vi "PRF_control.vi"(4 "PRF_Event Down":bool, 5 "mode selection":string(combo), 6 "error in (no error)":errorcluster, 7 "Input PRF":dbl, 8 "timeout (ms)":dbl=40000.0 format="%.2f", 9 "TCP from Orchid in":refnum<k5>) -> (0 "error out":errorcluster, 1 "PRF":dbl, 3 "connection ID out":refnum<k5>)   [LabVIEW 2016]
uses:
  TemperatureMeasure/Thermal_type.vi
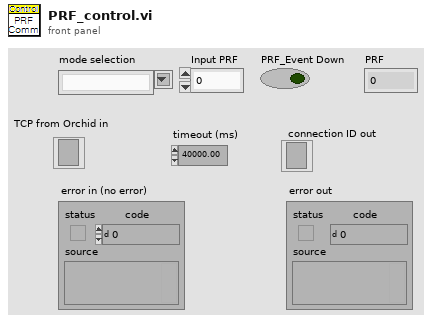
[diagram p1: front panel]
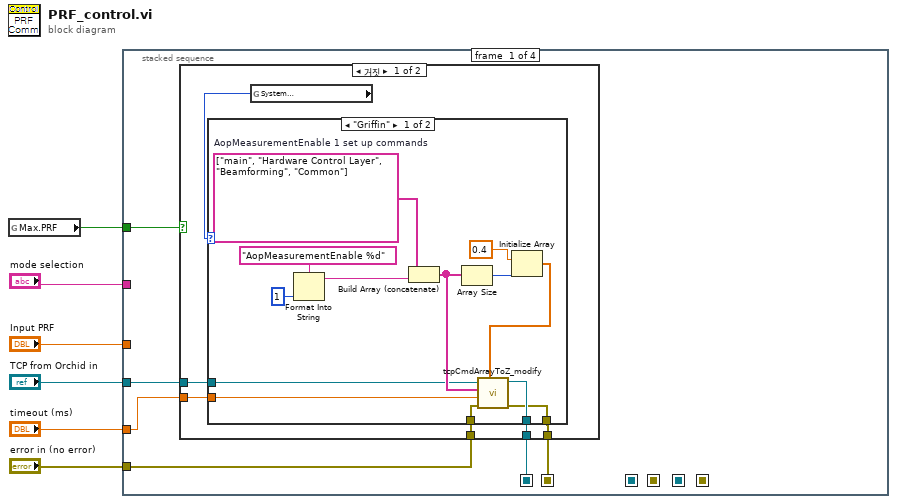
[diagram p0: block diagram]
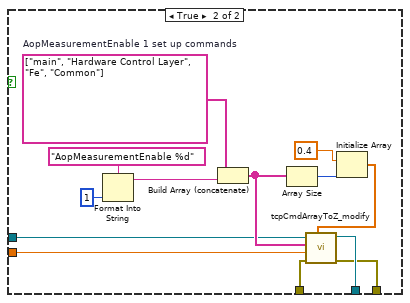
[diagram p3: hidden frame]
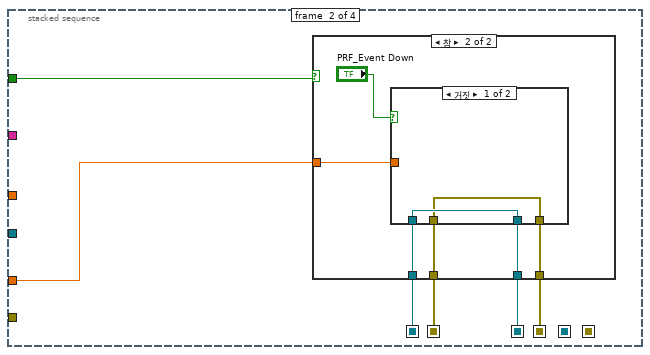
[diagram p4: hidden frame]
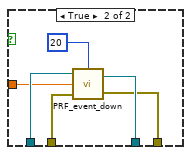
[diagram p6: hidden frame]
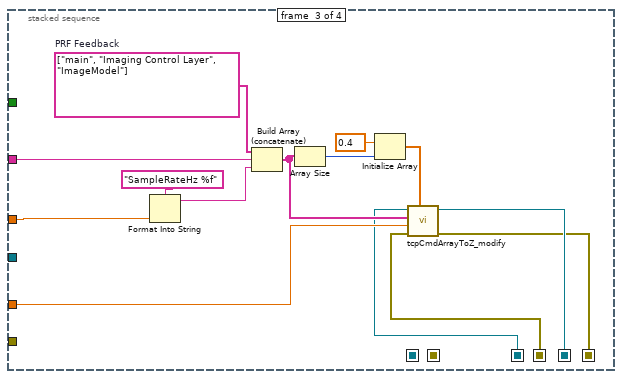
[diagram p7: hidden frame]
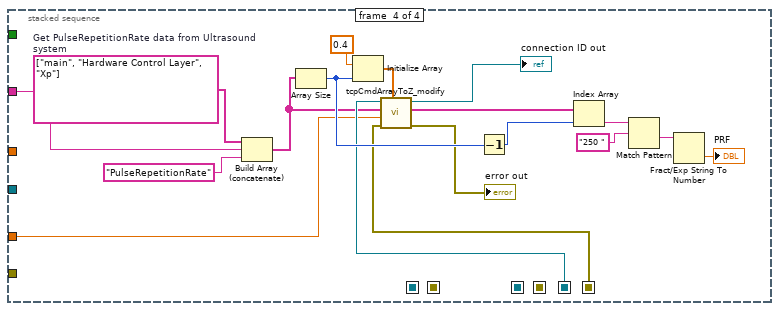
[diagram p8: hidden frame]
diagram:
  n1 = global read "Thermal_type.vi" "Max.PRF"() -> (w1:bool)
  n2 = stacked-sequence {
    seq-local: [w9 _ _ _] -> [_ w52 _ _]
    seq-local: [w8 _ _ _] -> [_ w51 _ _]
    seq-local: [_ w49 _ _] -> [_ _ w72 _]
    seq-local: [_ w48 _ _] -> [_ _ w71 _]
    seq-local: [_ _ w70 _] -> [_ _ _ w89]
    seq-local: [_ _ w69 _] -> [_ _ _ w87]
    tunnel: "mode selection" -> [_ _ w75 w85]
    tunnel: "Input PRF" -> [_ _ w74 _]
    tunnel: "TCP from Orchid in" -> [w12 _ _ _]
    tunnel: "timeout (ms)" -> [w10 w50 w73 w88]
    tunnel: "error in (no error)" -> [w11 _ _ _]
    tunnel: w1 -> [w7 w47 _ _]
    frame #0 {
      n3 = case shown="거짓" w7 {
        tunnel: w12 -> [w17 w38]
        tunnel: w11 -> [w16 w37]
        tunnel: w10 -> [w13 w36]
        tunnel: [w18 w35] -> w9
        tunnel: [w15 w34] -> w8
        frame False {
          n4 = global read "Thermal_type.vi" "System \nSelection"() -> (w14:enum32{"Common", "Frosk", "Griffin", "K2"})
          n5 = case shown="\"Griffin\"" w14 {
            tunnel: [w21 w33] -> w18
            tunnel: w17 -> [w23 w33]
            tunnel: [w20 w32] -> w15
            tunnel: w16 -> [w19 w32]
            tunnel: w13 -> [w22 _]
            frame "Griffin" {
              w31 = string[] ["main", "Hardware Control Layer", "Beamforming", "Common"]  # AopMeasurementEnable 1 set up commands
              n6 = Format Into String(format string="AopMeasurementEnable %d" ("Format String"), i8 1 ("입력 1")) -> (resulting string=w25:string)  [unwired: 2 in, 1 out]
              n7 = Build Array (concatenate)(w31, w25) -> (w30:string[])
              n8 = Array Size(array=w30) -> (size(s)=w29:i32)
              n9 = Initialize Array(0.4 ("원소"), w29) -> (w27:dbl[])
              n10 = call "tcpCmdArrayToZ_modify.vi"("Delay (sec)"=w27, "error in (no error)"=w19, "Timeout (ms)"=w22, "Command array"=w30, "connection ID in"=w23) -> ("error out"=w20:errorcluster, "connection ID out"=w21:refnum<k5>)  [unwired: 2 in, 3 out]
            }
            frame "Common", Default {
            }
          }
        }
        frame True {
          w46 = string[] ["main", "Hardware Control Layer", "Fe", "Common"]  # AopMeasurementEnable 1 set up commands
          n11 = Format Into String(format string="AopMeasurementEnable %d" ("Format String"), i8 1 ("입력 1")) -> (resulting string=w40:string)  [unwired: 2 in, 1 out]
          n12 = Build Array (concatenate)(w46, w40) -> (w45:string[])
          n13 = Array Size(array=w45) -> (size(s)=w44:i32)
          n14 = Initialize Array(0.4 ("원소"), w44) -> (w42:dbl[])
          n15 = call "tcpCmdArrayToZ_modify.vi"("Delay (sec)"=w42, "error in (no error)"=w37, "Timeout (ms)"=w36, "Command array"=w45, "connection ID in"=w38) -> ("error out"=w34:errorcluster, "connection ID out"=w35:refnum<k5>)  [unwired: 2 in, 3 out]
        }
      }
    }
    frame #1 {
      n16 = case shown="참" w47 {
        tunnel: w52 -> [w54 w60]
        tunnel: w51 -> [w53 w59]
        tunnel: w50 -> [_ w58]
        tunnel: [w54 w57] -> w49
        tunnel: [w53 w56] -> w48
        frame False {
        }
        frame True {
          n17 = case shown="거짓" "PRF_Event Down" {
            tunnel: w60 -> [w62 w68]
            tunnel: w59 -> [w61 w67]
            tunnel: w58 -> [_ w66]
            tunnel: [w62 w65] -> w57
            tunnel: [w61 w64] -> w56
            frame False {
            }
            frame True {
              n18 = call "PRF_event_down.vi"("Num_Down"=20, "error in (no error)"=w67, "Timeout (ms)"=w66, "connection ID out"=w68) -> ("error out"=w64:errorcluster, "connection ID out 2"=w65:refnum<k5>)
            }
          }
        }
      }
    }
    frame #2 {
      w81 = string[] ["main", "Imaging Control Layer", "ImageModel"]  # PRF Feedback
      n19 = Format Into String(format string="SampleRateHz %f" ("Format String"), w74) -> (resulting string=w76:string)  [unwired: 2 in, 1 out]
      n20 = Build Array (concatenate)(w81, w75, w76) -> (w82:string[])
      n21 = Array Size(array=w82) -> (size(s)=w80:i32)
      n22 = Initialize Array(0.4 ("element"), w80) -> (w78:dbl[])
      n23 = call "tcpCmdArrayToZ_modify.vi"("Delay (sec)"=w78, "error in (no error)"=w71, "Timeout (ms)"=w73, "Command array"=w82, "connection ID in"=w72) -> ("error out"=w69:errorcluster, "connection ID out"=w70:refnum<k5>)  [unwired: 2 in, 3 out]
    }
    frame #3 {
      w86 = string[] ["main", "Hardware Control Layer", "Xp"]  # Get PulseRepetitionRate data from Ultrasound system
      n24 = Build Array (concatenate)(w86, w85, "PulseRepetitionRate") -> (w83:string[])
      n25 = Array Size(array=w83) -> (size(s)=w97:i32)
      n26 = Initialize Array(0.4 ("원소"), w97) -> (w99:dbl[])
      n27 = call "tcpCmdArrayToZ_modify.vi"("Delay (sec)"=w99, "error in (no error)"=w87, "Timeout (ms)"=w88, "Command array"=w83, "connection ID in"=w89) -> ("error out"=→"error out":errorcluster, "Receive array"=w98:string[], "connection ID out"=→"connection ID out":refnum<k5>)  [unwired: 2 in, 2 out]
      n28 = Decrement(x=w97) -> (x-1=w95:i32)
      n29 = Index Array(array=w98, index=w95) -> (element=w96:string)
      n30 = Match Pattern(string=w96, regular expression="250 " ("정규식")) -> (after substring=w94:string)  [unwired: 1 in, 3 out]
      n31 = Fract/Exp String To Number(string=w94) -> (number=→"PRF":dbl)  [unwired: 3 in, 1 out]
    }
  }
